vi "串口参数断电保存全局变量.vi"() -> ()   [LabVIEW 2016, in "德润DR803L超标留样.lvlib"]
uses:
  <vilib>/Plasmionique/MB Master/MB_Master/MB_Master.lvclass
panel:
  out "流程中":bool
  out "超标留样信号":bool
  in  "CODCr超标浓度":dbl
  in  "CODMn超标浓度":dbl
  in  "总氮超标浓度":dbl
  in  "总磷超标浓度":dbl
  in  "氨氮超标浓度":dbl
  out "MB session in":refnum<class "MB_Master.lvclass">
  in  "MB通信方式选择":enum16{"串口", "TCP"}(ring)
  in  "PORT":string="1011"
  in  "IP":string="127.0.0.1"
  in  "Slave ID":u8=2
  in  "Serial Config":T1={"baud rate (bps)"=9600, "stop bits"=10, "parity"=0, "flow control"=0, "timeout"=1000, "retries"=1} {"stop bits" items=["1.0"=10, "1.5"=15, "2.0"=20]; "flow control" items=["None", "XON/XOFF", "RTS/CTS", "XON/XOFF & RTS/CTS", "DTR/DSR", "XON/XOFF & DTR/DSR"]; "parity" items=["None", "Odd", "Even", "Mark", "Space"]}
  in  "Error in":errorcluster
  in  "VISA resource name":refnum<visa-resource-name>="COM3" caption="VISA资源名称"
  # "MB串口参数"
  # "MBTCP参数"
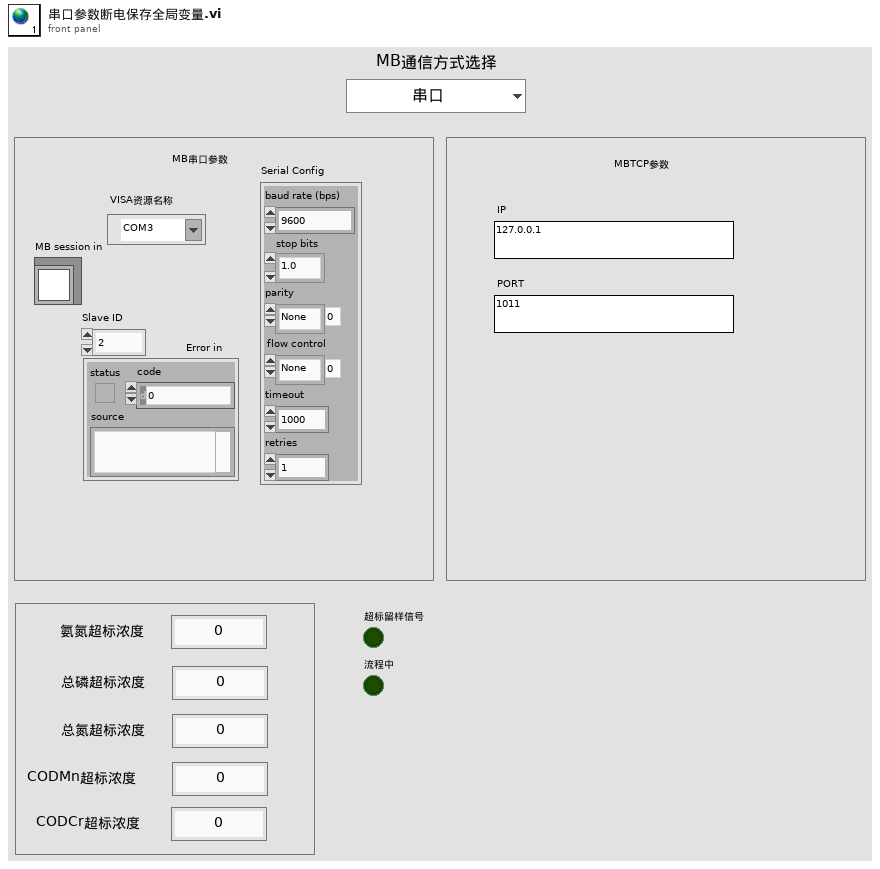
[diagram p1: front panel]
types:
  T1 = cluster{"baud rate (bps)":u32, "stop bits":u16, "parity":u16, "flow control":u16, "timeout":u32, "retries":i32}
diagram:
